vi "4.7.vi"() -> ()   [LabVIEW 2017]
panel:
  out "随机数":dbl
  out "次数":dbl
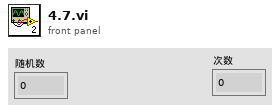
[diagram p1: front panel]
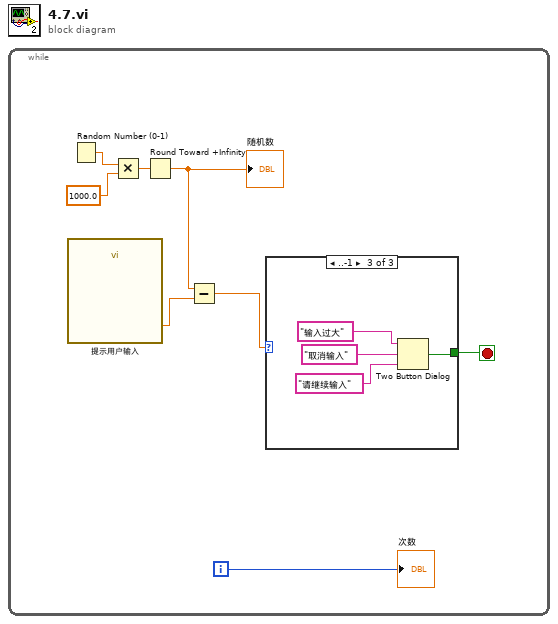
[diagram p0: block diagram]
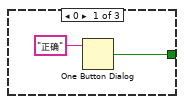
[diagram p2: hidden frame]
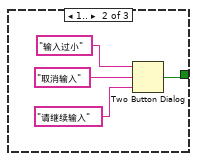
[diagram p3: hidden frame]
diagram:
  n1 = while {
    i -> [w5]
    stop <- w4 stop-if-true
    n2 = call "提示用户输入"() -> ("请输入1-1000"=w2:dbl)  [unwired: 17 in, 2 out]
    n3 = Random Number (0-1)() -> (number: 0 to 1=w7:dbl)
    n4 = Multiply(x=w7, y=1000.0) -> (x*y=w8:dbl)
    n5 = Round Toward +Infinity(x=w8) -> (ceil(x): smallest int >= x=w1:dbl)
    "随机数" <- w1
    n6 = Subtract(x=w1, y=w2) -> (x-y=w3:dbl)
    n7 = case shown="..-1" w3 {
      tunnel: [w9 w11 w15] -> w4
      frame 0 {
        n8 = One Button Dialog(message="正确") -> (true=w9:bool)  [unwired: 1 in]
      }
      frame 1.. {
        n9 = Two Button Dialog(message="输入过小", 1:"请继续输入", 2:"取消输入") -> (T button?=w11:bool)
      }
      frame ..-1 {
        n10 = Two Button Dialog(message="输入过大", 1:"请继续输入", 2:"取消输入") -> (T button?=w15:bool)
      }
    }
    "次数" <- w5
  }
